vi "GlobalXyData.vi"() -> ()   [LabVIEW 2014]
panel:
  in  "XChName(XY)":string[](array[string])
  in  "ChName(XY)":string[](array[string])
  in  "XYグラフ(Nプロット)":cluster{"X配列":dbl[], "Y配列":dbl[]}[](array[cluster])
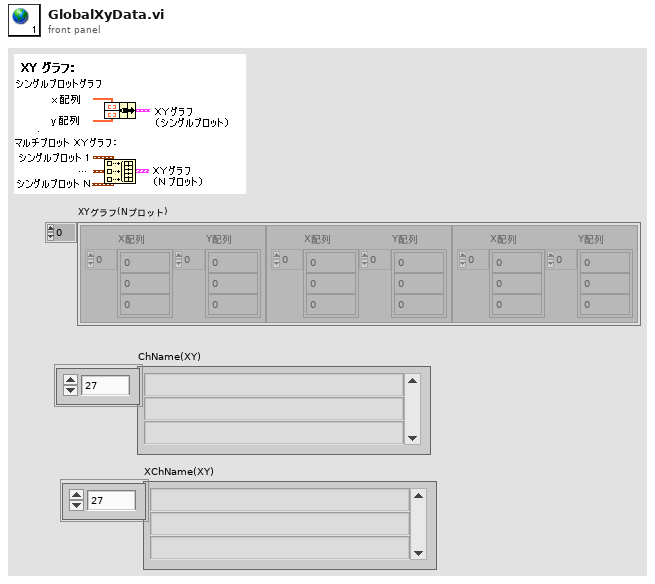
[diagram p1: front panel]
diagram:
